vi "NodesApp.vi"() -> ()   [LabVIEW 2021]
panel:
  out "Node Values":dbl[](array[numeric])
  in  "GetValue":bool
  in  "Stop":bool
  out "error out":errorcluster
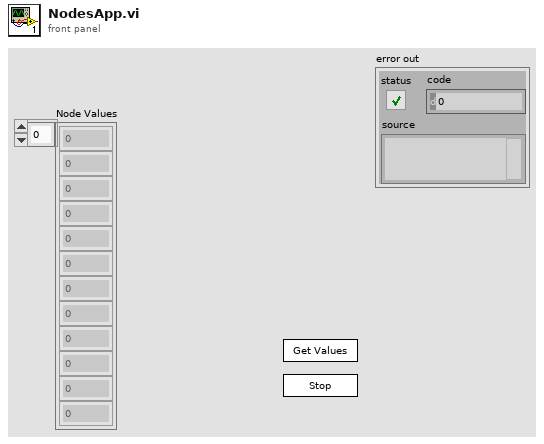
[diagram p1: front panel]
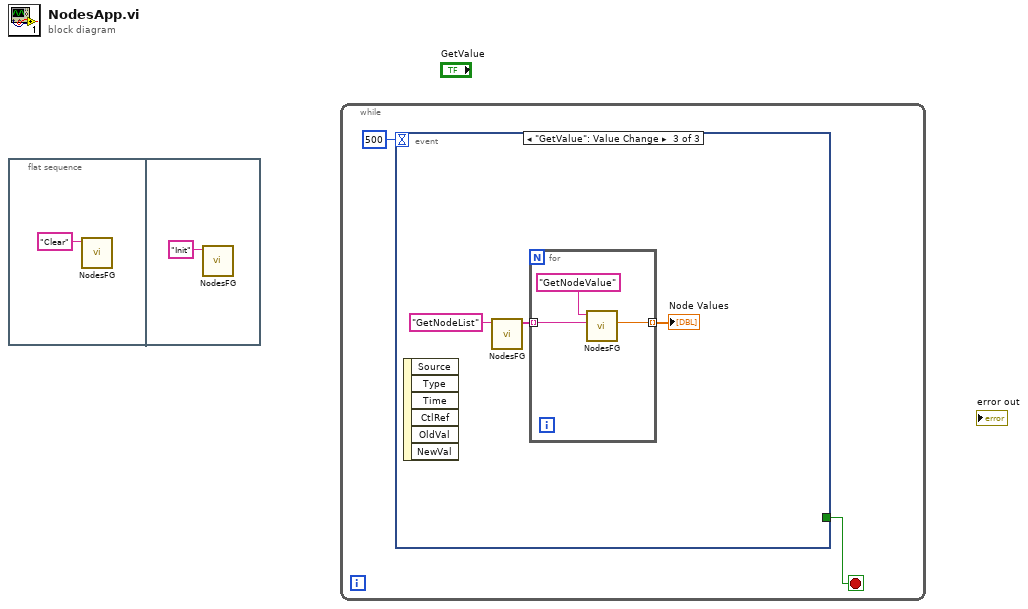
[diagram p0: block diagram]
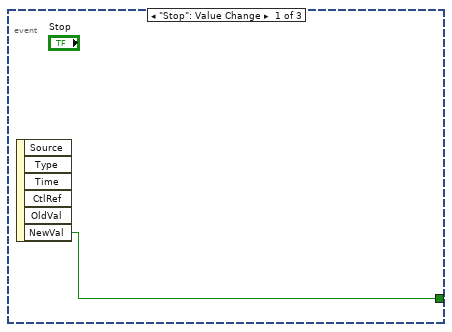
[diagram p2: hidden frame]
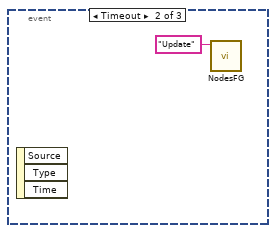
[diagram p3: hidden frame]
diagram:
  n1 = flat-sequence {
    frame #0 {
      n2 = call "NodesFG.vi"("Function"="Clear") -> ()  [unwired: 8 in, 3 out]
    }
    frame #1 {
      n3 = call "NodesFG.vi"("Function"="Init") -> ()  [unwired: 8 in, 3 out]
    }
  }
  n4 = while {
    stop <- w4 stop-if-true
    n5 = event shown="[2] \"GetValue\": Value Change" {
      selector: _ -> [_ _ _]
      dyn-events: _ -> [_ _ _]
      timeout: 500 -> [_ _ _]
      tunnel: [w5 _ _] -> w4
      event "Stop": Value Change {
        n6 = event-data() -> ("NewVal"=w5:bool)  [unwired: 1 in, 5 out]
      }
      event Timeout {
        n7 = event-data() -> ()  [unwired: 1 in, 3 out]
        n8 = call "NodesFG.vi"("Function"="Update") -> ()  [unwired: 8 in, 3 out]
      }
      event "GetValue": Value Change {
        n9 = event-data() -> ()  [unwired: 1 in, 6 out]
        n10 = call "NodesFG.vi"("Function"="GetNodeList") -> ("Node List"=w8:string[])  [unwired: 8 in, 2 out]
        n11 = for {
          tunnel: w8 -> [w11] mode=indexing
          tunnel: [w10] -> w7 mode=indexing
          n12 = call "NodesFG.vi"("Node Name"=w11, "Function"="GetNodeValue") -> ("Value"=w10:dbl)  [unwired: 7 in, 2 out]
        }
        "Node Values" <- w7
      }
    }
  }
